vi "roi_to_txt.vi"(8 "error in":errorcluster, 10 "path in":path, 11 "output array in":T1(array[cluster])) -> (0 "error out":errorcluster)   [LabVIEW 2010, in "TrajectoryMH100122AODRAPS.lvclass"]
uses:
  TrajectoryMH100122AODRAPS.lvclass
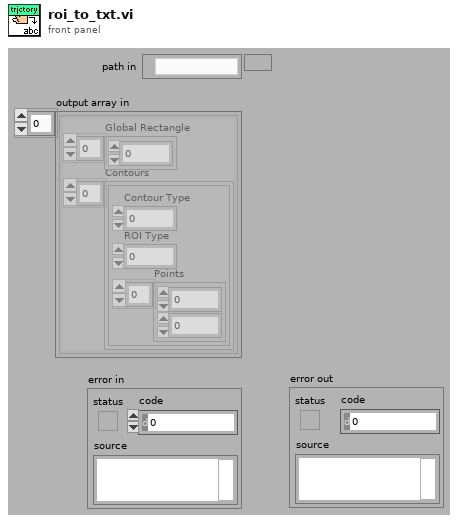
[diagram p1: front panel]
types:
  T1 = cluster{"Global Rectangle":i32[], "Contours":cluster{"Contour Type":u32, "ROI Type":u32, "Points":i32[]}[]}[]
  T2 = enum16{"open", "replace", "create", "open or create", "replace or create", "replace or create with confirmation"}
  T3 = cluster{"Contour Type":u32, "ROI Type":u32, "Points":i32[]}[]
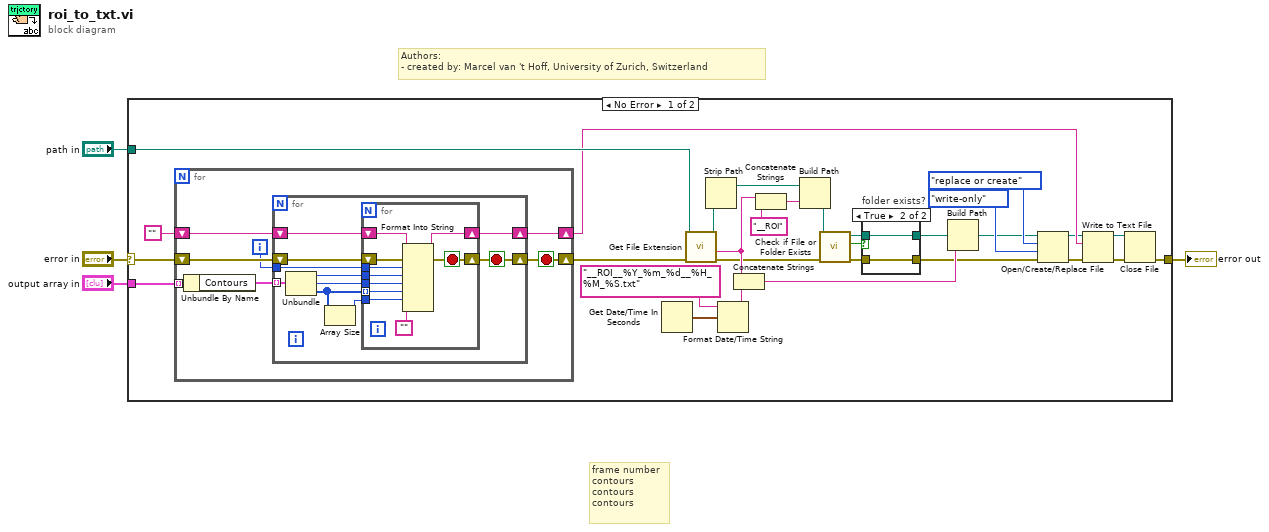
[diagram p0: block diagram]
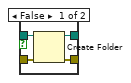
[diagram p2: hidden frame]
diagram:
  # "frame number\ncontours\ncontours\ncontours"
  # "Authors: \n- created by: Marcel van 't Hoff, University of Zurich, Switzerland"
  n1 = case shown="No Error" "error in" {
    selector: "error in" -> [w33 w68]
    tunnel: "output array in" -> [w24 _]
    tunnel: [w20 w68] -> w3
    tunnel: "path in" -> [w30 _]
    frame No Error {
      n2 = for {
        tunnel: w24 -> [w47] mode=indexing
        shift-right: [w46] -> w29
        shift-left: "" -> [w45]
        shift-right: [w41] -> w10
        shift-left: w33 -> [w44]
        i -> [w43]
        stop <- w41 stop-if-true
        n3 = Unbundle By Name(w47) -> ("Contours"=w42:T3)
        n4 = for {
          tunnel: w42 -> [w57] mode=indexing
          shift-right: [w54] -> w46
          shift-left: w45 -> [w53]
          tunnel: w43 -> [w51]
          shift-right: [w48] -> w41
          shift-left: w44 -> [w52]
          stop <- w48 stop-if-true
          n5 = Unbundle(w57) -> ("Contour Type"=w55:u32, "ROI Type"=w56:u32, "Points"=w50:i32[])
          n6 = Array Size(array=w50) -> (size(s)=w49:i32)
          n7 = for {
            tunnel: w50 -> [w67] mode=indexing
            tunnel: w56 -> [w61]
            tunnel: w55 -> [w62]
            shift-right: [w66] -> w54
            shift-left: w53 -> [w65]
            tunnel: w51 -> [w63]
            tunnel: w49 -> [w59]
            shift-right: [w58] -> w48
            shift-left: w52 -> [w64]
            stop <- w58 stop-if-true
            n8 = Format Into String(initial string=w65, error in=w64, w63, w62, w61, w67, w59, "" ("input 4")) -> (resulting string=w66:string, error out=w58:errorcluster)  [unwired: 1 in]
          }
        }
      }
      n9 = Get Date/Time In Seconds() -> (seconds since 1Jan1904=w22:timestamp)
      n10 = call <vilib>:"Get File Extension.vi"("error in (no error)"=w10, "file"=w30) -> ("error out"=w8:errorcluster, "filename without extension"=w13:string, "dup file"=w19:path)  [unwired: 6 in, 1 out]
      n11 = Strip Path(path=w19) -> (stripped path=w16:path)  [unwired: 1 out]
      n12 = Format Date/Time String(time format string (%c)="__ROI__%Y_%m_%d__%H_%M_%S.txt", seconds (now)=w22) -> (date/time string=w21:string)  [unwired: 1 in]
      n13 = Concatenate Strings(w13, w21) -> (w18:string)
      n14 = Concatenate Strings(w13, "__ROI" ("name or relative path")) -> (w11:string)
      n15 = Build Path(base path=w16, name or relative path=w11) -> (appended path=w9:path)
      n16 = call <vilib>:"Check if File or Folder Exists.vi"("error in (no error)"=w8, "path"=w9) -> ("error out"=w7:errorcluster, "file or folder exists?"=w5:bool, "dup path"=w6:path)  [unwired: 7 in]
      n17 = case "folder exists?" shown="True" w5 {
        tunnel: [w38 w39] -> w17
        tunnel: [w37 w40] -> w15
        tunnel: w7 -> [w36 w39]
        tunnel: w6 -> [w35 w40]
        frame False {
          n18 = Create Folder(path (use dialog)=w35, error in=w36) -> (created path=w37:path, error out=w38:errorcluster)  [unwired: 1 in, 1 out]
        }
        frame True {
        }
      }
      n19 = Build Path(base path=w15, name or relative path=w18) -> (appended path=w14:path)
      n20 = Open/Create/Replace File(file path (use dialog)=w14, error in=w17, operation (0:open)=T2."replace or create", access (0:read/write)=enum16{"read/write", "read-only", "write-only"}."write-only") -> (refnum out=w27:refnum<file>, error out=w28:errorcluster)  [unwired: 2 in, 1 out]
      n21 = Write to Text File(file (use dialog)=w27, text=w29, error in=w28) -> (refnum out=w25:refnum<file>, error out=w26:errorcluster)  [unwired: 1 in, 1 out]
      n22 = Close File(refnum=w25, error in=w26) -> (error out=w20:errorcluster)  [unwired: 1 out]
    }
    frame Error {
    }
  }
  "error out" <- w3
